vi "Log Reference.vi"(7 "Action":T1, 10 "Global Log Reference":refnum<data-value>) -> (2 "Global Log Reference out":refnum<data-value>)   [LabVIEW 2016, in "Stream Log.lvlib" / "Global Application Log.lvclass"]
doc: "--\nCopyright © 2017 Composed SystemsI All rights reserved.\n\nAuthor: Jon McBee <jon.mcbee@composed.io>\n\nThis library is provided \"AS IS\" ,WITHOUT WARRANTIES OR\nCONDITIONS OF ANY KIND, either express or implied.\n\nComposed Systems -- composed.io\n\nStream 0.0.1.1\nJon McBee - Composed Systems\nCopyright (c) 2017, Composed Systems"
uses:
  <userlib>/Composed Systems/Stream/Log/Global Application Log/Global Application Log.lvclass
  <userlib>/Composed Systems/Stream/Log/Global Application Log/Log Reference Action.ctl
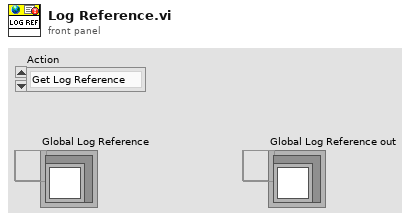
[diagram p1: front panel]
types:
  T1 = typedef "Stream Log.lvlib/Global Application Log.lvclass/Log Reference Action.ctl" = enum16{"Get Log Reference", "Set Log Reference"}
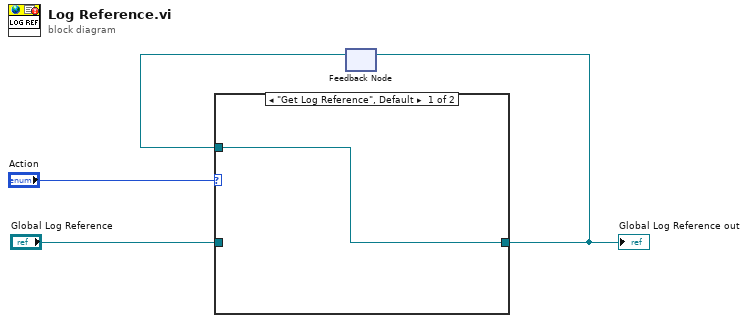
[diagram p0: block diagram]
diagram:
  n1 = feedback #1() -> (w2:refnum<data-value>)  [unwired: 1 in]
  n2 = case shown="\"Get Log Reference\", Default" "Action" {
    tunnel: w2 -> [w5 _]
    tunnel: [w5 w6] -> w3
    tunnel: "Global Log Reference" -> [_ w6]
    frame "Get Log Reference", Default {
    }
    frame "Set Log Reference" {
    }
  }
  "Global Log Reference out" <- w3
  n3 = feedback-in #1(w3) -> ()
